vi "DFD Plot MRate Freq Response.vi"(5 "output option":u16(ring) items=["Auto", "Floating-Point Only", "Fixed-Point Only"], 6 "fs in [Hz]":dbl=-1.0, 7 "# freq bins":i32=-1, 8 "error in (no error)":errorcluster, 9 "dB on? (T)":bool=TRUE, 10 "phase view":T6, 11 "multirate filter in":T1={"mMRate_Structure"=enum."IIR", "mMRate_Mode"=0, "mMRate_Factor"=-1, "mMRate_FIRParams"={"mMRate_FIR_H"=[], "mMRate_FIR_IsNyquist?"=FALSE, "mMRate_FIR_IsSymmetric?"=FALSE}, "mMRate_CICParams"={"mMRate_CIC_#Stage"=0, "mMRate_CIC_Lag"=0, "mMRate_CIC_Type"=enum."Lowpass"}, "mMRate_Order"=0, "mMRate_Version"="2.0", "mMRate_Comments"="", "mMRate_RationalFactor"={"mMRate_L"=-1, "mMRate_M"=-1}, "mMRate_Fs"=1.0, "mMRate_Quantized?"=FALSE, "mMRate_QFilterGain"=1.0, "mMRate_CoefWl"=16, "mMRate_Scaling"={"mMRate_ScaleByPowerOf2?"=FALSE, "mMRate_ScaleType"=enum."No Norm"}, "mMRate_InputWl"=16, "mMRate_OutputWl"=16, "mMRate_OutputMode"=enum."Truncation", "mMRate_MultMode"=enum."Truncated", "mMRate_BitPruning"=FALSE, "mMRate_GainWl"=16, "mMRate_OutputFwl"=0, "mMRate_SumIwl"=0, "mMRate_InputIwl "=16, "mMRate_SumWl"=32, "mMRate_CoefIwl"=0} {"mMRate_SumWl" min=1 max=32 step=1; "mMRate_InputIwl" min=1 max=32 step=1; "mMRate_GainWl" min=1 max=32 step=1; "mMRate_OutputWl" min=1 max=32 step=1; "mMRate_InputWl" min=1 max=32 step=1; "mMRate_CoefWl" min=1 max=32 step=1; "mMRate_Mode" items=["Default"=-1, "No Rate Change"=0, "Interpolation"=1, "Decimation"=2, "Interpolated"=3, "Rational"=4]}) -> (0 "error out":errorcluster, 1 "phase response":cluster{"f0":dbl, "df":dbl, "values":dbl[]}[](graph), 2 "magnitude response":cluster{"f0":dbl, "df":dbl, "values":dbl[]}[](graph), 3 "multirate filter out":T1={"mMRate_Structure"=enum."IIR", "mMRate_Mode"=0, "mMRate_Factor"=-1, "mMRate_FIRParams"={"mMRate_FIR_H"=[], "mMRate_FIR_IsNyquist?"=FALSE, "mMRate_FIR_IsSymmetric?"=FALSE}, "mMRate_CICParams"={"mMRate_CIC_#Stage"=0, "mMRate_CIC_Lag"=0, "mMRate_CIC_Type"=enum."Lowpass"}, "mMRate_Order"=0, "mMRate_Version"="2.0", "mMRate_Comments"="", "mMRate_RationalFactor"={"mMRate_L"=-1, "mMRate_M"=-1}, "mMRate_Fs"=1.0, "mMRate_Quantized?"=FALSE, "mMRate_QFilterGain"=1.0, "mMRate_CoefWl"=16, "mMRate_Scaling"={"mMRate_ScaleByPowerOf2?"=FALSE, "mMRate_ScaleType"=enum."No Norm"}, "mMRate_InputWl"=16, "mMRate_OutputWl"=16, "mMRate_OutputMode"=enum."Truncation", "mMRate_MultMode"=enum."Truncated", "mMRate_BitPruning"=FALSE, "mMRate_GainWl"=16, "mMRate_OutputFwl"=0, "mMRate_SumIwl"=0, "mMRate_InputIwl "=16, "mMRate_SumWl"=32, "mMRate_CoefIwl"=0} {"mMRate_SumWl" min=1 max=32 step=1; "mMRate_InputIwl" min=1 max=32 step=1; "mMRate_GainWl" min=1 max=32 step=1; "mMRate_OutputWl" min=1 max=32 step=1; "mMRate_InputWl" min=1 max=32 step=1; "mMRate_CoefWl" min=1 max=32 step=1; "mMRate_Mode" items=["Default"=-1, "No Rate Change"=0, "Interpolation"=1, "Decimation"=2, "Interpolated"=3, "Rational"=4]})   [LabVIEW 2017, in "NI_DigFilterLicensed.lvlib"]
doc: "Plots the frequency responses, including the magnitude and phase responses, of multirate filters."
uses:
  <vilib>/addons/Digital Filter Design/NI_DigFilterLicensed.lvlib
  <vilib>/addons/Digital Filter Design/_Objects.llb/DFD Multirate Filter Obj.ctl
  <vilib>/addons/Digital Filter Design/_Objects.llb/DFD Multirate Mode.ctl
  <vilib>/addons/Digital Filter Design/_Objects.llb/DFD Coef Norm Type.ctl
  <vilib>/addons/Digital Filter Design/_Objects.llb/DFD Round-off Mode.ctl
  <vilib>/addons/Digital Filter Design/_Objects.llb/DFD FXP MRate Multiply Mode.ctl
  <vilib>/addons/Digital Filter Design/_Objects.llb/DFD Phase Setting.ctl
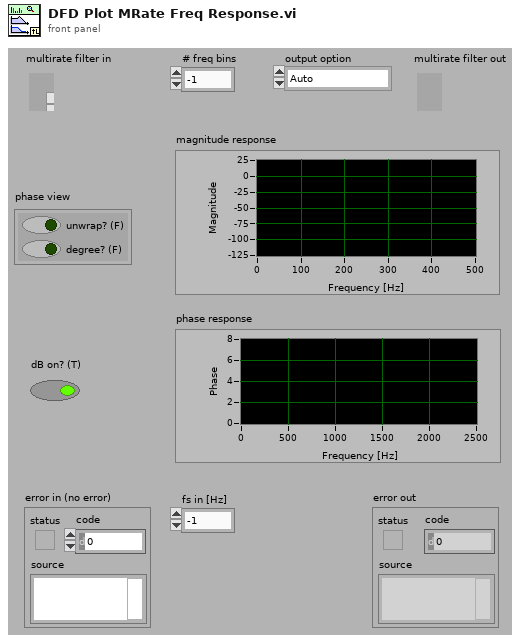
[diagram p1: front panel]
types:
  T1 = typedef "NI_DigFilterLicensed.lvlib/DFD Multirate Filter Obj.ctl" = cluster{"mMRate_Structure":enum16{"CIC", "FIR", "IIR", "Lattice"}, "mMRate_Mode":T2, "mMRate_Factor":i32, "mMRate_FIRParams":cluster{"mMRate_FIR_H":dbl[], "mMRate_FIR_IsNyquist?":bool, "mMRate_FIR_IsSymmetric?":bool}, "mMRate_CICParams":cluster{"mMRate_CIC_#Stage":i32, "mMRate_CIC_Lag":i32, "mMRate_CIC_Type":enum16{"Lowpass", "Highpass"}}, "mMRate_Order":i32, "mMRate_Version":string, "mMRate_Comments":string, "mMRate_RationalFactor":cluster{"mMRate_L":i32, "mMRate_M":i32}, "mMRate_Fs":dbl, "mMRate_Quantized?":bool, "mMRate_QFilterGain":dbl, "mMRate_CoefWl":i16, "mMRate_Scaling":cluster{"mMRate_ScaleByPowerOf2?":bool, "mMRate_ScaleType":T3}, "mMRate_InputWl":i16, "mMRate_OutputWl":i16, "mMRate_OutputMode":T4, "mMRate_MultMode":T5, "mMRate_BitPruning":bool, "mMRate_GainWl":i16, "mMRate_OutputFwl":i16, "mMRate_SumIwl":i16, "mMRate_InputIwl ":i16, "mMRate_SumWl":i16, "mMRate_CoefIwl":i16}
  T2 = typedef "NI_DigFilterLicensed.lvlib/DFD Multirate Mode.ctl" = i16
  T3 = typedef "NI_DigFilterLicensed.lvlib/DFD Coef Norm Type.ctl" = enum16{"No Norm", "Time Domain 1-Norm", "Time Domain 2-Norm", "Time Domain Inf-Norm"}
  T4 = typedef "NI_DigFilterLicensed.lvlib/DFD Round-off Mode.ctl" = enum16{"Nearest", "Truncation"}
  T5 = typedef "NI_DigFilterLicensed.lvlib/DFD FXP MRate Multiply Mode.ctl" = enum16{"Truncated", "Full"}
  T6 = typedef "NI_DigFilterLicensed.lvlib/DFD Phase Setting.ctl" = cluster{"unwrap? (F)":bool, "degree? (F)":bool}
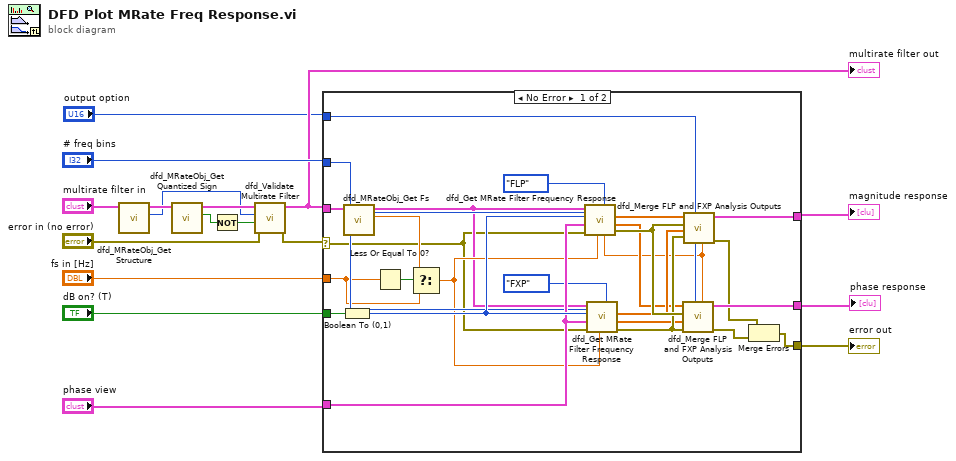
[diagram p0: block diagram]
diagram:
  n1 = call <vilib>:"dfd_MRateObj_Get Structure.vi"("multirate filter in"="multirate filter in") -> ("structure"=w1:enum16{"CIC", "FIR", "IIR", "Lattice"}, "dup multirate filter"=w2:T1)  [unwired: 9 out]
  n2 = call <vilib>:"dfd_MRateObj_Get Quantized Sign.vi"("multirate filter in"=w2) -> ("is Quantized?"=w5:bool, "dup multirate filter"=w6:T1)  [unwired: 9 out]
  n3 = Not(x=w5) -> (.not. x?=w4:bool)
  n4 = call <vilib>:"dfd_Validate Multirate Filter.vi"("error in (no error)"="error in (no error)", "skip FXP? (T)"=w4, "preferred structure"=w1, "multirate filter in"=w6) -> ("error out"=w3:errorcluster, "multirate filter out"=w12:T1)  [unwired: 6 out]
  "multirate filter out" <- w12
  n5 = case shown="No Error" w3 {
    selector: w3 -> [w19 w44]
    tunnel: "# freq bins" -> [w38 _]
    tunnel: "phase view" -> [w39 _]
    tunnel: "dB on? (T)" -> [w43 _]
    tunnel: w12 -> [w23 _]
    tunnel: "fs in [Hz]" -> [w25 _]
    tunnel: [w30 w44] -> w13
    tunnel: "output option" -> [w31 _]
    tunnel: [w28 _] -> w9
    tunnel: [w27 _] -> w8
    frame No Error {
      n6 = Boolean To (0,1)(Boolean=w43) -> (0, 1=w40:i16)
      n7 = call <vilib>:"dfd_MRateObj_Get Fs.vi"("multirate filter in"=w23) -> ("fs"=w21:dbl, "dup multirate filter"=w22:T1)  [unwired: 9 out]
      n8 = Less Or Equal To 0?(x=w25) -> (x <= 0?=w26:bool)
      n9 = Select(t=w21, s=w26, f=w25) -> (s? t:f=w24:dbl)
      n10 = call <vilib>:"dfd_Get MRate Filter Frequency Response.vi"("type (FLP)"=enum16{"FLP", "FXP"}."FLP", "fs in [Hz]"=w24, "# freq bins (auto)"=w38, "error in"=w19, "phase view"=w39, "magnitude"=w40, "multirate filter out"=w22) -> ("error out"=w36:errorcluster, "phase"=w32:dbl[], "magnitude"=w41:dbl[], "df"=w18:dbl)  [unwired: 1 out]
      n11 = call <vilib>:"dfd_Get MRate Filter Frequency Response.vi"("type (FLP)"=enum16{"FLP", "FXP"}."FXP", "fs in [Hz]"=w24, "# freq bins (auto)"=w38, "error in"=w19, "phase view"=w39, "magnitude"=w40, "multirate filter out"=w22) -> ("error out"=w34:errorcluster, "phase"=w33:dbl[], "magnitude"=w35:dbl[])  [unwired: 2 out]
      n12 = call <vilib>:"dfd_Merge FLP and FXP Analysis Outputs.vi"("delta"=w18, "output option"=w31, "error in FXP"=w34, "response FXP"=w33, "error in FLP"=w36, "response FLP"=w32) -> ("error out"=w29:errorcluster, "freq responses"=w27:cluster{"f0":dbl, "df":dbl, "values":dbl[]}[])  [unwired: 4 out]
      n13 = call <vilib>:"dfd_Merge FLP and FXP Analysis Outputs.vi"("delta"=w18, "output option"=w31, "error in FXP"=w34, "response FXP"=w35, "error in FLP"=w36, "response FLP"=w41) -> ("error out"=w20:errorcluster, "freq responses"=w28:cluster{"f0":dbl, "df":dbl, "values":dbl[]}[])  [unwired: 4 out]
      n14 = Merge Errors(w20, w29) -> (w30:errorcluster)
    }
    frame Error {
    }
  }
  "error out" <- w13
  "phase response" <- w8
  "magnitude response" <- w9
